vi "Read TagDistanceArray.vi"(8 "error in (no error)":errorcluster, 11 "Anchor in":refnum<class "Anchor.lvclass">) -> (0 "error out":errorcluster, 2 "TagDistanceArray":T1(array[cluster]), 3 "Anchor out":refnum<class "Anchor.lvclass">)   [LabVIEW 2014, in "Anchor.lvclass"]
uses:
  Anchor.lvclass
  Tag.lvclass
  Anchor.lvclass/Anchor.ctl
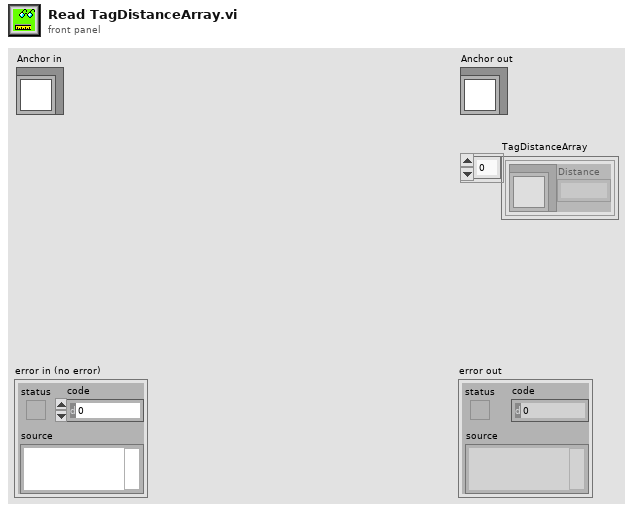
[diagram p1: front panel]
types:
  T1 = cluster{"Tag.lvclass":refnum<class "Tag.lvclass">, "Distance":dbl}[]
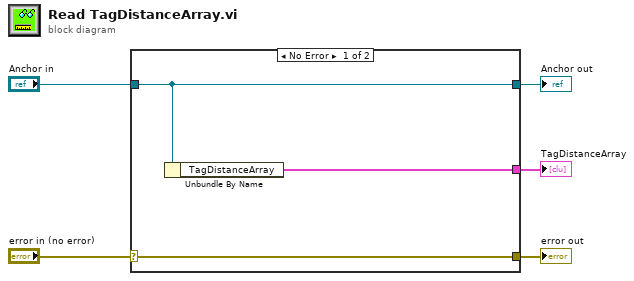
[diagram p0: block diagram]
diagram:
  n1 = case shown="No Error" "error in (no error)" {
    selector: "error in (no error)" -> [w8 w9]
    tunnel: [w8 w9] -> w4
    tunnel: [w7 w10] -> w2
    tunnel: "Anchor in" -> [w7 w10]
    tunnel: [w6 _] -> w1
    frame No Error {
      n2 = Unbundle By Name(w7) -> ("TagDistanceArray"=w6:T1)
    }
    frame Error {
    }
  }
  "error out" <- w4
  "Anchor out" <- w2
  "TagDistanceArray" <- w1
